vi "Test.vi"() -> ()   [LabVIEW 2024]
uses:
  Config Files Management/section data--cluster.ctl
  Config Files Management/API Config Files.lvlib
panel:
  out "restitucion":T1
  out "despues borrado":T1
  out "antes borrado":T1
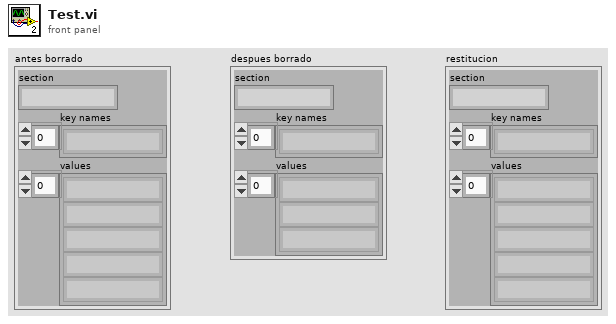
[diagram p1: front panel]
types:
  T1 = typedef "API Config Files.lvlib/section data--cluster.ctl" = cluster{"section":string, "key names":string[], "values":string[]}
  T2 = typedef "NI_LVConfig.lvlib/Config Data RefNum.ctl" = refnum<k1>
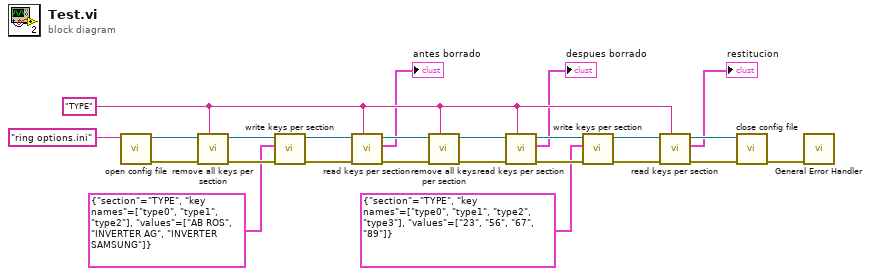
[diagram p0: block diagram]
diagram:
  w9 = "TYPE" ("section")
  n1 = call "open config file.vi"("file name"="ring options.ini") -> ("error out"=w13:errorcluster, "Refnum out"=w12:T2)  [unwired: 8 in, 1 out]
  n2 = call "remove all keys per section.vi"("section"=w9, "error in (no error)"=w13, "Refnum in"=w12) -> ("error out"=w10:errorcluster, "Refnum out"=w11:T2)  [unwired: 7 in]
  n3 = call "write keys per section.vi"("error in (no error)"=w10, "section data"=T1 {"section"="TYPE", "key names"=["type0", "type1", "type2"], "values"=["AB ROS", "INVERTER AG", "INVERTER SAMSUNG"]}, "Refnum in"=w11) -> ("error out"=w8:errorcluster, "Refnum out"=w4:T2)  [unwired: 7 in]
  n4 = call "read keys per section.vi"("section"=w9, "error in (no error)"=w8, "Refnum in"=w4) -> ("error out"=w23:errorcluster, "section data"=→"antes borrado":T1, "Refnum out"=w22:T2)  [unwired: 6 in]
  n5 = call "remove all keys per section.vi"("section"=w9, "error in (no error)"=w23, "Refnum in"=w22) -> ("error out"=w21:errorcluster, "Refnum out"=w19:T2)  [unwired: 7 in]
  n6 = call "read keys per section.vi"("section"=w9, "error in (no error)"=w21, "Refnum in"=w19) -> ("error out"=w18:errorcluster, "section data"=→"despues borrado":T1, "Refnum out"=w17:T2)  [unwired: 6 in]
  n7 = call "write keys per section.vi"("error in (no error)"=w18, "section data"=T1 {"section"="TYPE", "key names"=["type0", "type1", "type2", "type3"], "values"=["23", "56", "67", "89"]}, "Refnum in"=w17) -> ("error out"=w16:errorcluster, "Refnum out"=w15:T2)  [unwired: 7 in]
  n8 = call "read keys per section.vi"("section"=w9, "error in (no error)"=w16, "Refnum in"=w15) -> ("error out"=w20:errorcluster, "section data"=→"restitucion":T1, "Refnum out"=w6:T2)  [unwired: 6 in]
  n9 = call "close config file.vi"("error in (no error)"=w20, "Refnum in"=w6) -> ("error out"=w24:errorcluster)  [unwired: 9 in]
  n10 = call <vilib>:"General Error Handler.vi"("error in (no error)"=w24) -> ()  [unwired: 10 in, 5 out]
